vi "FPGA DDS DC IP.vi"(9 "Signal Amplitude (x 2^15)":u16=32768) -> (2 "Accumulator Value":u32 format="%.3e", 3 "Signal Value":i16)   [LabVIEW 2013, in "IRIO.lvlib"]
uses:
  IRIO.lvlib
  <vilib>/rvi/Arithmetic/AddSubMult/XNode/nirviSatArithmetic.xnode
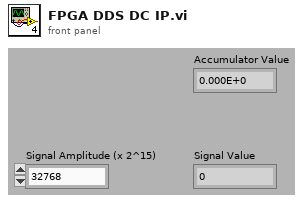
[diagram p1: front panel]
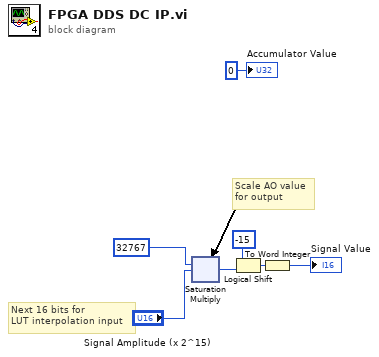
[diagram p0: block diagram]
diagram:
  # "Scale AO value\nfor output"
  # "Next 16 bits for\nLUT interpolation input"
  n1 = xnode ("Saturation Multiply")("x"=i16 32767 ("Accumulator Value"), "y"="Signal Amplitude (x 2^15)") -> ("x*y"=w5:i32)
  n2 = Logical Shift(y=-15, x=w5) -> (x << y=w7:i32)
  n3 = To Word Integer(number=w7) -> (16bit integer=→"Signal Value":i16)
  "Accumulator Value" <- u32 0 ("Accumulator Value")
